vi "Report&Trace.vi"() -> ()   [LabVIEW 2020]
uses:
  Global_Variable/Global.vi
panel:
  in  "判定结果":bool[][](array[boolean])=[[TRUE]]
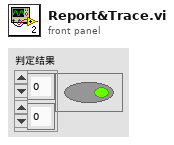
[diagram p1: front panel]
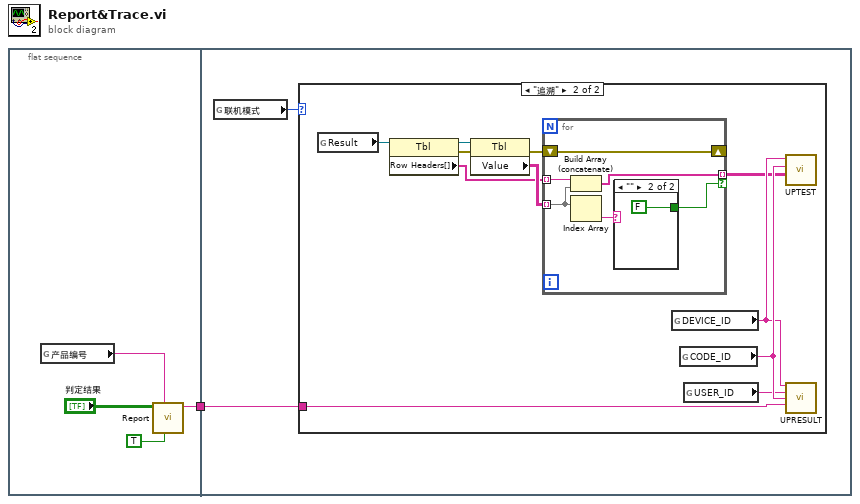
[diagram p0: block diagram]
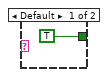
[diagram p3: hidden frame]
diagram:
  n1 = flat-sequence {
    tunnel: [w2] -> w1
    tunnel: w1 -> [w6]
    frame #0 {
      n2 = global read "Global.vi" "产品编号"() -> (w5:string)
      n3 = call "Report.vi"("文件重命名"=TRUE, "文件名称"=w5, "检测结果"="判定结果") -> ("PRODUCT_VAULE"=w2:string)  [unwired: 7 in, 1 out]
    }
    frame #1 {
      n4 = global read "Global.vi" "联机模式"() -> (w7:enum16{"单机", "追溯"})
      n5 = case shown="\"追溯\"" w7 {
        tunnel: w6 -> [_ w8]
        frame "单机", Default {
        }
        frame "追溯" {
          n6 = global read "Global.vi" "Result"() -> (w10:refnum<vi>)
          n7 = property class="Tbl"(reference=w10) -> (reference out=w15:refnum<vi>, error out=w12:errorcluster, "Row Headers[]"=w13:string[])  [unwired: 1 in]
          n8 = property class="Tbl"(reference=w15, error in=w12) -> (error out=w11:errorcluster, "Value"=w14:string[][])  [unwired: 1 out]
          n9 = for {
            tunnel: w14 -> [w22] mode=indexing
            tunnel: w13 -> [w23] mode=indexing
            tunnel: [w20] -> w9 mode=indexing if=w21
            shift-right: [w19] -> _
            shift-left: w11 -> [w19]
            n10 = Build Array (concatenate)(w23, w22) -> (w20:string[])
            n11 = Index Array(array=w22) -> (element=w24:string)  [unwired: 1 in]
            n12 = case shown="\"\"" w24 {
              tunnel: [TRUE FALSE] -> w21
              frame Default {
              }
              frame "" {
              }
            }
          }
          n13 = global read "追溯Global.vi" "DEVICE_ID"() -> (w17:string)
          n14 = global read "追溯Global.vi" "CODE_ID"() -> (w18:string)
          n15 = global read "追溯Global.vi" "USER_ID"() -> (w16:string)
          n16 = call "UPTEST.vi"("Result"=w9, "CODE_ID"=w18, "DEVICE_ID"=w17) -> ()  [unwired: 6 in, 1 out]
          n17 = call "UPRESULT.vi"("DEVICE_ID"=w17, "USER_ID"=w16, "CODE_ID"=w18, "RESULT_VALUE"=w8) -> ()  [unwired: 11 in, 1 out]
        }
      }
    }
  }
